vi "Add.vi"() -> ()   [LabVIEW 2018]
panel:
  in  "B":i32=6
  in  "A":i32=5
  out "C":i32
  # "+"
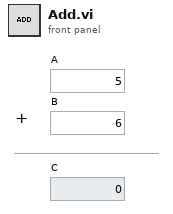
[diagram p1: front panel]
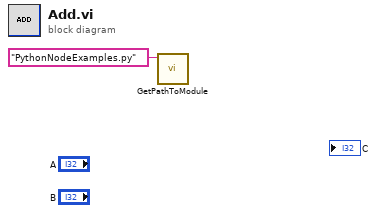
[diagram p0: block diagram]
diagram:
  n1 = call "GetPathToModule.vi"("module name"="PythonNodeExamples.py") -> ()  [unwired: 10 in, 1 out]
